vi "RGmove2.vi"(2 "delay before read (ms)":u32=50, 3 "Grating, gr/mm":u16(ring)=2 items=["2400", "1800", "1200", "600", "300", "150"], 4 "Wavelength, nm":dbl=10.0 format="%.3f") -> (1 "error?":bool)   [LabVIEW 2017]
doc: "The Advanced Serial Read and Write example performs a Serial Port Read, a Serial Port Write, or a combination of these actions while setting some advanced serial features like buffer size, termination characters, and XON/XOFF flow control. The user selects the actions (read or write) on the front panel. If both are selected, the VI will write the data first, read the data and then close the VISA session that is opened to the port. \n\nThe parameters set for the serial port must match the parameters of the connected instrument or device. In this example, the bytes to read parameter specifies the number of bytes that the serial port reads. If there were more bytes at the port than the number specified in bytes to read, those bytes would not be read. Also, if you specify to read more bytes than the number of bytes actually read, you might receive a timeout error message.\n\nINSTRUCTIONS:\n1) Select the serial resource and configuration parameters (baud rate, data bits, parity, stop bits, flow control).\n2) Termination character can be enabled and set. Also, set the required input buffer size prior to running the example.\n3) Select the operations to be performed. \n4) Connect the serial port to your device. If no device is available, perform a loopback test by doing one of the following. Short pins 2 and 3 on a RS-232 cable or short pin 4 to pin 8 and pin 5 to pin 9 on a RS-485/422 cable. \n5) Run the VI to see the data read. (The \"read string\" will match the \"string to write\" if a loopback test was performed.)\n\nThis example exposes several advanced features that you may need for your application. Not all applications need all the features shown in this example. The input buffer size is likely an important setting that you want to control in your application. This example expands upon the flow control option for XON and XOFF, allowing the user to choose those control characters. The timeout parameter has been brought to the front panel so a user can specify the time period the VISA Read will wait for the number of bytes to read before timing out. Also, the user has several controls for the termination character, which is discussed later.\n\nNote that you can press the write and read buttons and change the bytes to read parameters on the fly, while the example is running. However, you must stop the example to change the other configuration parameters after the example has started running, and then run again.\n\nSet the I/O buffer size slightly higher the amount of data you expect to receive. This is very important for applications that don't use flow control, as you may lose characters if the receive buffer overflows.\n\nSetting the timeout period ensures that the operation returns with a timeout error if the operation cannot be performed in the specified time period. \n\nSome devices require a termination character in order to identify the end of command strings. Some devices send a termination character to signify the end of data to be read. \n\nThis example shows how you can end the Read operation once a termination character is detected in the buffer and/or append a termination character at the end of the Write data. To enable the Read to end on a termination character, use the VISA Configure Serial Port or use the VISA Properties Serial End Mode for Reads, Termination Character Enable, and Termination Character. To end the Write with a termination character, use the VISA Properties Serial End Mode for Writes, the Send End Enable, and Termination Character. In this example, the same termination character is used for both the Read and the Write. You can specify two different characters for your application, if desired.\n\nYour application may require specific characters for the XON/XOFF Flow Control. You can specify these characters with the VISA Properties Flow Control XOFF Character and Flow Control XON Character. Note that if the standard XON and XOFF characters are used, then decimal 17 and 19 are unavailable for data values. Remember that using flow control and setting an adequate buffer size allow you to prevent buffer overflows."
uses:
  Monochromator.lvlib
  global_Test.vi
  <vilib>/Utility/error.llb/DialogType.ctl
panel:
  out "code out":i32 format="%0.0f"
  out "move":bool
  out "delay":bool
  out "move done":bool
  out "bytes to read":u32
  out "string 2":string="\n"
  out "Loop":i32
  in  "stop":bool
  # "Move Wavelength"
  # "nm"
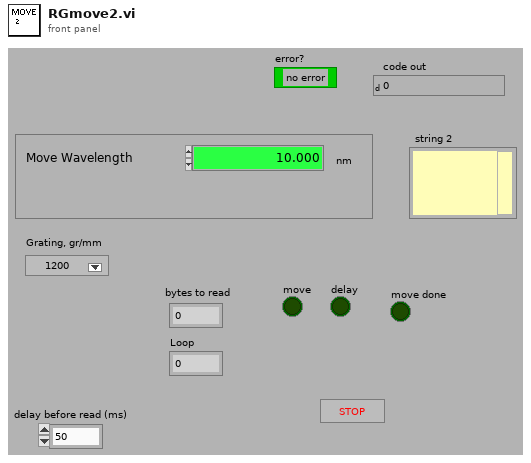
[diagram p1: front panel]
types:
  T1 = typedef "DialogType.ctl" = u16
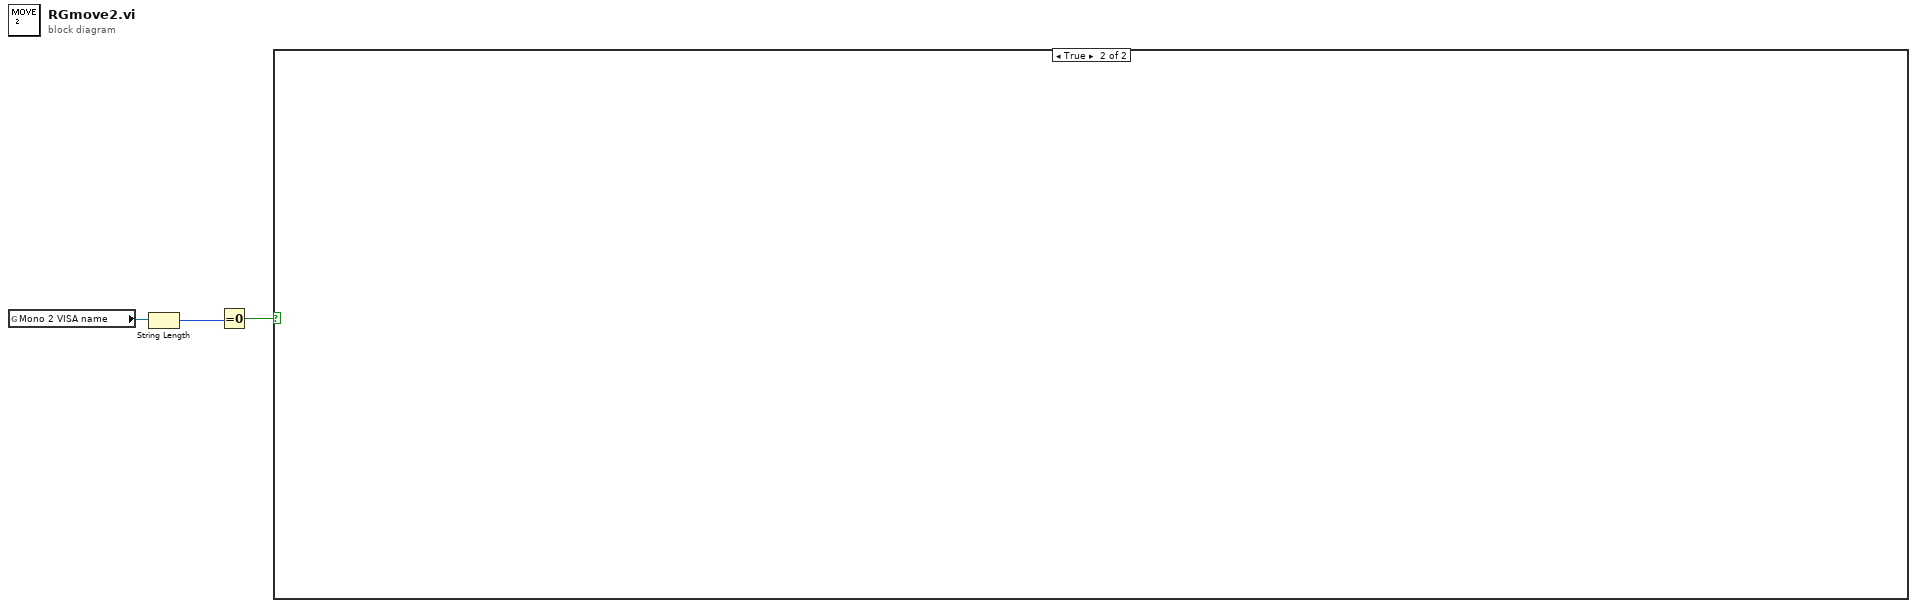
[diagram p0: block diagram]
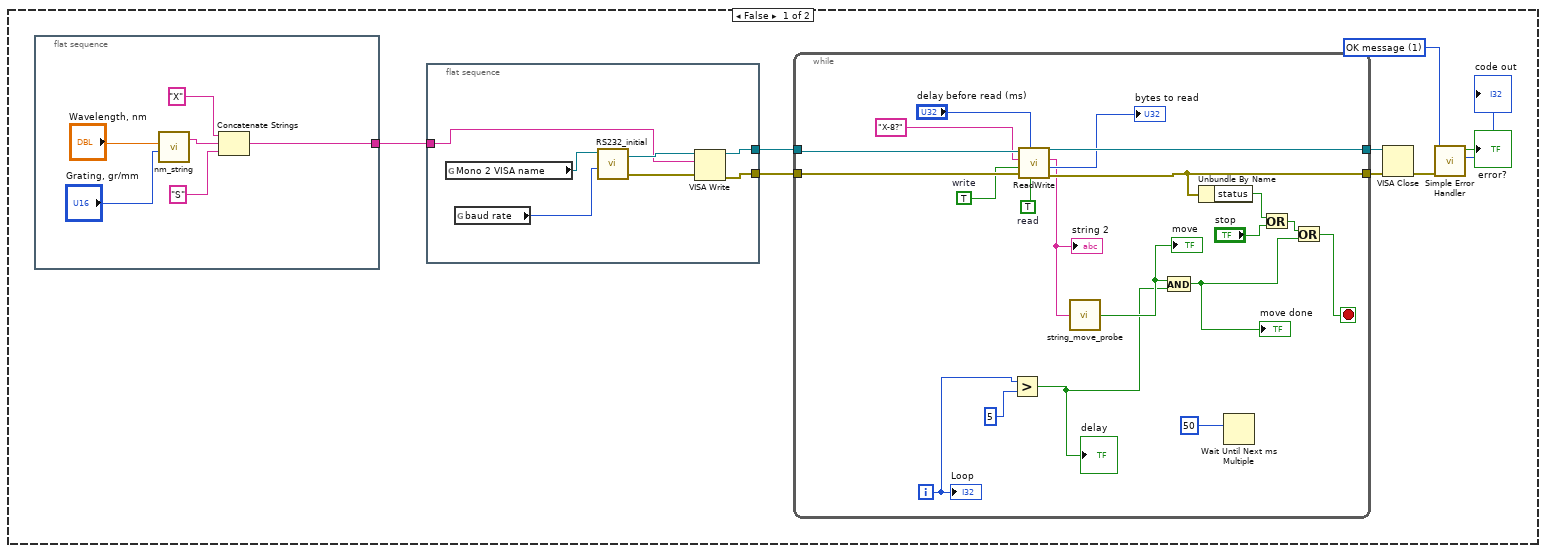
[diagram p2: hidden frame]
diagram:
  n1 = global read "global_Test.vi" "Mono 2 VISA name"() -> (w1:refnum<visa-resource-name>)
  n2 = String Length(string=w1) -> (length=w3:i32)
  n3 = Equal To 0?(x=w3) -> (x = 0?=w2:bool)
  n4 = case shown="True" w2 {
    frame False {
      w5 = T1 1 items=["no dialog", "OK message", "continue or stop message", "OK message + warnings", "continue/stop + warnings"] ("type of dialog (OK msg:1)")
      n5 = flat-sequence {
        tunnel: [w13] -> w7
        frame #0 {
          n6 = call "nm_string.vi"("Grating, gr/mm"="Grating, gr/mm", "Wavelength, nm"="Wavelength, nm") -> ("nm_String"=w16:string)  [unwired: 2 in, 1 out]
          n7 = Concatenate Strings("X" ("string"), w16, "S" ("string")) -> (w13:string)
        }
      }
      n8 = flat-sequence {
        tunnel: [w25] -> w9
        tunnel: [w24] -> w8
        tunnel: w7 -> [w21]
        frame #0 {
          n9 = global read "global_Test.vi" "Mono 2 VISA name"() -> (w20:refnum<visa-resource-name>)
          n10 = global read "global_Test.vi" "baud rate"() -> (w19:u16)
          n11 = call "RS232_initial.vi"("baud rate"=w19, "VISA resource name"=w20) -> ("error out"=w22:errorcluster, "VISA name out"=w23:refnum<visa-resource-name>)  [unwired: 2 in]
          n12 = VISA Write(VISA resource name=w23, write buffer=w21, error in (no error)=w22) -> (VISA resource name out=w25:refnum<visa-resource-name>, error out=w24:errorcluster)  [unwired: 1 out]
        }
      }
      n13 = while {
        tunnel: [w45] -> w11
        tunnel: [w44] -> w10
        tunnel: w9 -> [w40]
        tunnel: w8 -> [w39]
        i -> [w31]
        stop <- w37 stop-if-true
        w33 = TRUE  # read
        w35 = TRUE  # write
        n14 = Greater?(x=w31, y=5 ("x")) -> (0:w26:bool)
        "delay" <- w26
        n15 = call "ReadWrite.vi"("read"=w33, "delay before read (ms)"="delay before read (ms)", "error in"=w39, "write"=w35, "string to write"="X-8?", "VISA  name in"=w40) -> ("error out"=w44:errorcluster, "bytes to read"=→"bytes to read":u32, "read string"=w29:string, "VISA out"=w45:refnum<visa-resource-name>)
        "string 2" <- w29
        n16 = call "string_move_probe.vi"("read string 2"=w29) -> ("move"=w27:bool)
        "move" <- w27
        n17 = And(x=w27, y=w26) -> (x .and. y?=w28:bool)
        "move done" <- w28
        n18 = Unbundle By Name(w44) -> ("status"=w43:bool)
        n19 = Wait Until Next ms Multiple(millisecond multiple=u32 50) -> ()  [unwired: 1 out]
        n20 = Or(x=w43, y="stop") -> (x .or. y?=w38:bool)
        n21 = Or(x=w38, y=w28) -> (x .or. y?=w37:bool)
        "Loop" <- w31
      }
      n22 = VISA Close(VISA resource name=w11, error in (no error)=w10) -> (error out=w12:errorcluster)
      n23 = call <vilib>:"Simple Error Handler.vi"("type of dialog (OK msg:1)"=w5, "error in (no error)"=w12) -> ("error?"=→"error?":bool, "code out"=→"code out":i32)  [unwired: 3 in, 3 out]
    }
    frame True {
    }
  }
